vi "Create DUT Setup Parameters.vi"(8 "error in (no error)":errorcluster, 11 "QPA Measurement in":refnum<class "QPA Measurement.lvclass">) -> (0 "error out":errorcluster, 2 "DUT Setup Parameters":string[](array[string]), 3 "QPA Measurement out":refnum<class "QPA Measurement.lvclass">)   [LabVIEW 2016, in "QPA Measurement.lvlib" / "QPA Measurement.lvclass"]
uses:
  QPA Measurement.lvclass
  C:/Projects/STS/Common/Sequence Automation/Plugins/Measurement Interface.lvlibp/Measurement Interface.lvclass
  QPA Measurement.lvclass/QPA Measurement.ctl
  Protected Methods/Read DUT Setup Parameters.vi
  Plugins/Measurement Interface.lvlibp/Private Methods/Measurement Parameters/Read Measurement Parameters.vi
  Plugins/String Database.lvlibp/String Database.lvclass
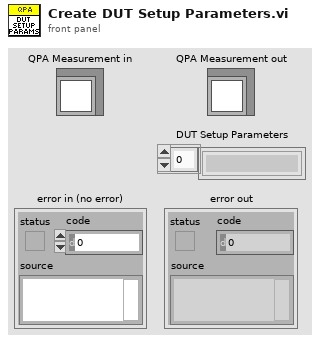
[diagram p1: front panel]
types:
  T1 = typedef "QPA Measurement.lvlib/QPA Measurement.lvclass/Parameter.ctl" = cluster{"Name":string, "PropertyObject Type":enum16{"Container", "String", "Boolean", "Number", "NamedType", "Reference", "Array", "Aperture Time"}}
  T2 = enum16{"Container", "String", "Boolean", "Number", "NamedType", "Reference", "Array", "Aperture Time"}
  T3 = typedef "QPA MSMT Waveform Manager.lvclass/RF Waveform.ctl" = cluster{"Name":string, "Path":path, "Headroom":dbl, "Burst Length":dbl}
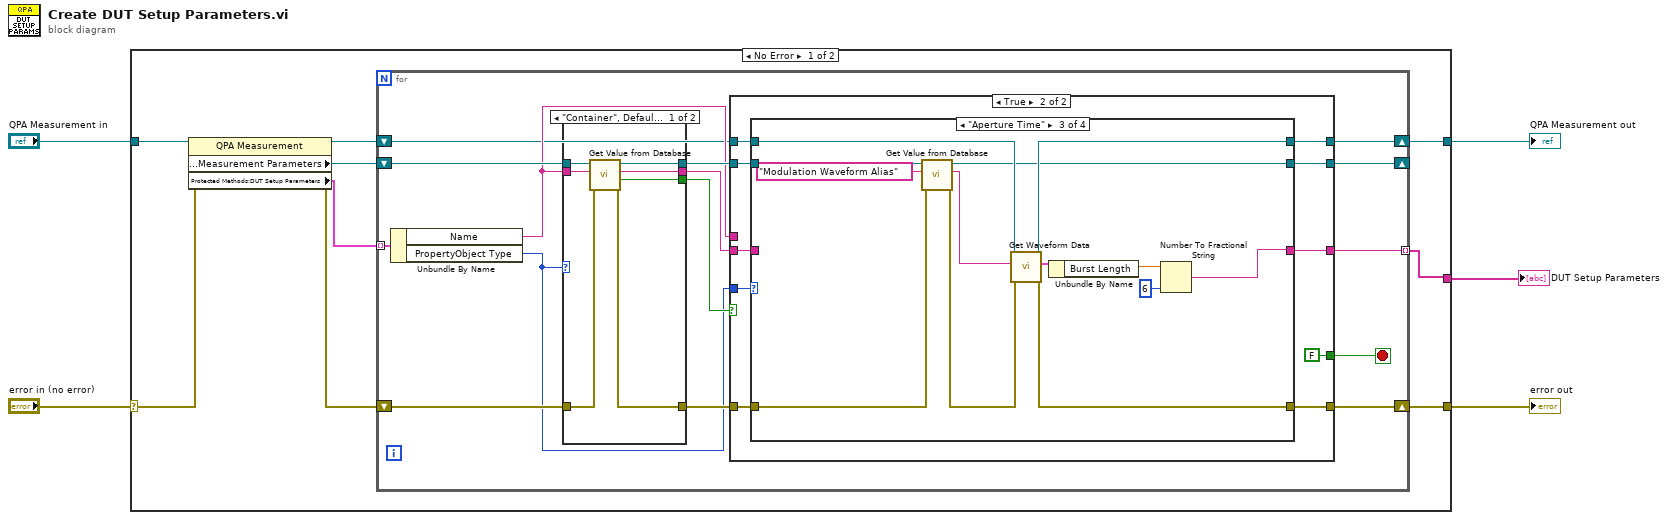
[diagram p0: block diagram]
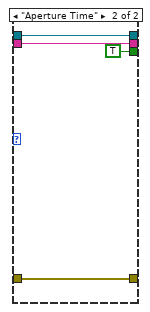
[diagram p2: hidden frame]
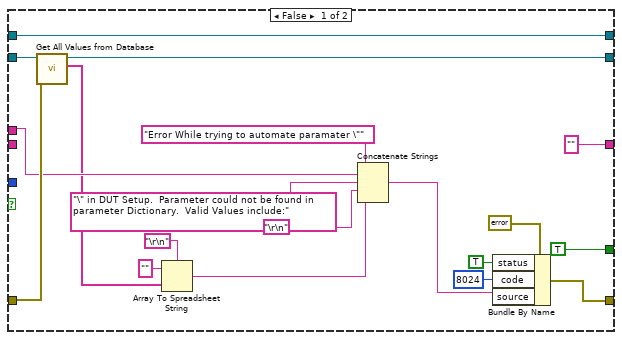
[diagram p3: hidden frame]
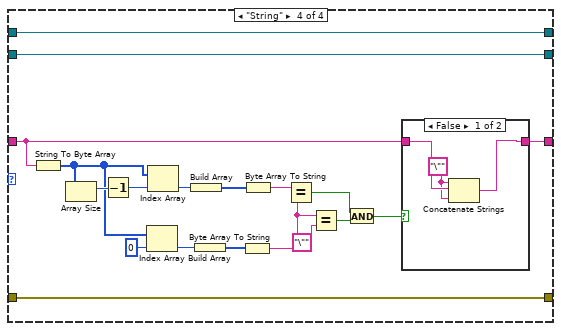
[diagram p6: hidden frame]
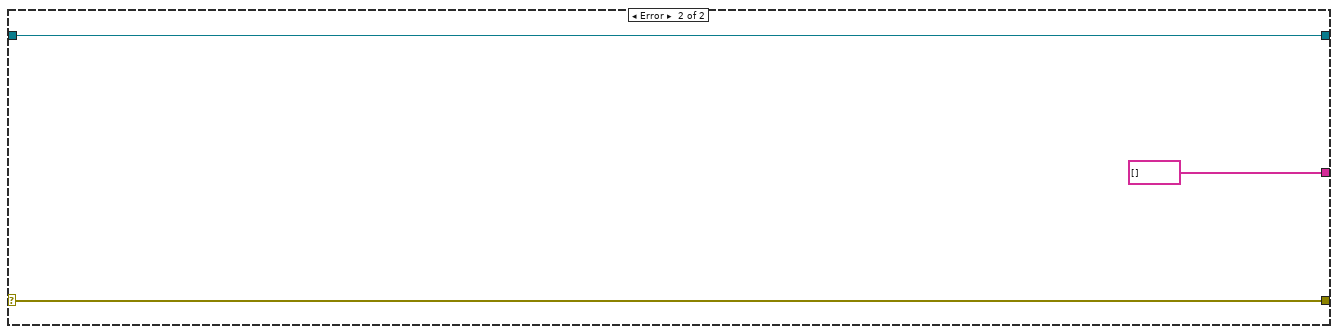
[diagram p8: hidden frame]
diagram:
  n1 = case shown="No Error" "error in (no error)" {
    selector: "error in (no error)" -> [w14 w116]
    tunnel: [w8 w116] -> w4
    tunnel: [w6 w115] -> w2
    tunnel: "QPA Measurement in" -> [w13 w115]
    tunnel: [w9 string[] []] -> w1
    frame No Error {
      n2 = property class="QPA Measurement"(reference=w13, error in=w14) -> (reference out=w7:refnum<class "QPA Measurement.lvclass">, error out=w11:errorcluster, "Protected Methods:Measurement Parameters"=w10:refnum<class "String Database.lvclass">, "Protected Methods:DUT Setup Parameters"=w12:T1[])
      n3 = for {
        tunnel: w12 -> [w29] mode=indexing
        shift-right: [w23] -> w8
        shift-left: w11 -> [w28]
        shift-right: [w21] -> _
        shift-left: w10 -> [w27]
        tunnel: [w24] -> w9 mode=indexing
        shift-right: [w16] -> w6
        shift-left: w7 -> [w17]
        stop <- w19 stop-if-true
        n4 = Unbundle By Name(w29) -> ("Name"=w18:string, "PropertyObject Type"=w15:T2)
        n5 = case shown="\"Container\", Default" w15 {
          tunnel: w28 -> [w36 w38]
          tunnel: w27 -> [w35 w40]
          tunnel: [w34 w39] -> w26
          tunnel: [w33 TRUE ("Entry Found")] -> w25
          tunnel: [w32 w38] -> w22
          tunnel: [w31 w40] -> w20
          tunnel: w18 -> [w30 w39]
          frame "Container", Default {
            n6 = call "Get Value from Database.vi"("error in (no error)"=w36, "Entry Name"=w30, "Message in"=w35) -> ("error out"=w32:errorcluster, "Entry Found"=w33:bool, "Entry Value"=w34:string, "Message out"=w31:refnum<class "String Database.lvclass">)  [unwired: 5 in]
          }
          frame "Aperture Time" {
          }
        }
        n7 = case shown="True" w25 {
          tunnel: w15 -> [_ w69]
          tunnel: w26 -> [_ w68]
          tunnel: ["" ("Entry Value") w67] -> w24
          tunnel: [w59 w64] -> w23
          tunnel: w22 -> [w49 w65]
          tunnel: [w50 w63] -> w21
          tunnel: w20 -> [w51 w62]
          tunnel: [TRUE ("status") FALSE ("status")] -> w19
          tunnel: w18 -> [w43 _]
          tunnel: w17 -> [w41 w61]
          tunnel: [w41 w60] -> w16
          frame False {
            n8 = call "Get All Values from Database.vi"("error in (no error)"=w49, "String Database in"=w51) -> ("Names"=w42:string[], "String Database out"=w50:refnum<class "String Database.lvclass">)  [unwired: 6 in, 2 out]
            n9 = Array To Spreadsheet String(delimiter (Tab)="\r\n", array=w42, 3:"" ("format string")) -> (spreadsheet string=w46:string)
            n10 = Concatenate Strings("Error While trying to automate paramater \"", w43, "\" in DUT Setup.  Parameter could not be found in parameter Dictionary.  Valid Values include:" ("string"), "\r\n", w46) -> (w53:string)
            n11 = Bundle By Name(cluster=errorcluster {"status"=FALSE, "code"=0, "source"=""} ("error out"), "status"=TRUE, "code"=8024, "source"=w53) -> (w59:errorcluster)
          }
          frame True {
            n12 = case shown="\"Aperture Time\"" w69 {
              tunnel: w68 -> [w73 w77 _ w94]
              tunnel: [w73 w77 w87 w95] -> w67
              tunnel: w65 -> [w72 w76 w84 w93]
              tunnel: [w72 w76 w86 w93] -> w64
              tunnel: [w71 w75 w79 w92] -> w63
              tunnel: w62 -> [w71 w75 w85 w92]
              tunnel: w61 -> [w70 w74 w81 w91]
              tunnel: [w70 w74 w80 w91] -> w60
              frame "Container", Default {
              }
              frame "Number" {
              }
              frame "Aperture Time" {
                n13 = call "Get Value from Database.vi"("error in (no error)"=w84, "Entry Name"="Modulation Waveform Alias", "Message in"=w85) -> ("error out"=w83:errorcluster, "Entry Value"=w82:string, "Message out"=w79:refnum<class "String Database.lvclass">)  [unwired: 5 in, 1 out]
                n14 = call "Get Waveform Data.vi"("error in (no error)"=w83, "Waveform to Retrieve"=w82, "QPA Measurement in"=w81) -> ("error out"=w86:errorcluster, "RF Waveform"=w90:T3, "QPA Measurement out"=w80:refnum<class "QPA Measurement.lvclass">)  [unwired: 6 in]
                n15 = Unbundle By Name(w90) -> ("Burst Length"=w89:dbl)
                n16 = Number To Fractional String(number=w89, precision (6)=i16 6) -> (F-format string=w87:string)  [unwired: 2 in]
              }
              frame "String" {
                n17 = String To Byte Array(string=w94) -> (unsigned byte array=w107:u8[])
                n18 = Array Size(array=w107) -> (size(s)=w109:i32)
                n19 = Decrement(x=w109) -> (x-1=w108:i32)
                n20 = Index Array(array=w107, index=0) -> (element=w105:u8)
                n21 = Index Array(array=w107, index=w108) -> (element=w106:u8)
                n22 = Build Array(w106) -> (w103:u8[])
                n23 = Build Array(w105) -> (w104:u8[])
                n24 = Byte Array To String(unsigned byte array=w104) -> (string=w101:string)
                n25 = Byte Array To String(unsigned byte array=w103) -> (string=w102:string)
                n26 = Equal?(x=w102, y=w101) -> (x = y?=w98:bool)
                n27 = Equal?(x=w101, y="\"") -> (x = y?=w99:bool)
                n28 = And(x=w98, y=w99) -> (x .and. y?=w96:bool)
                n29 = case shown="False" w96 {
                  tunnel: [w111 w113] -> w95
                  tunnel: w94 -> [w112 w113]
                  frame False {
                    w110 = "\"" ("string")
                    n30 = Concatenate Strings(w110, w112, w110) -> (w111:string)
                  }
                  frame True {
                  }
                }
              }
            }
          }
        }
      }
    }
    frame Error {
    }
  }
  "error out" <- w4
  "QPA Measurement out" <- w2
  "DUT Setup Parameters" <- w1
